vi "Main.vi"() -> ()   [LabVIEW 2019]
uses:
  <vilib>/myRIO/Common/Instrument Driver Framework/myRIO v1.0/UART/vis/myRIO v1.0 Close UART.vi
  <vilib>/Utility/error.llb/Error Cluster From Error Code.vi
  <vilib>/myRIO/Common/Instrument Driver Framework/Utilities/vis/FPGA Ref Manager.vi
  <vilib>/myRIO/Common/Instrument Driver Framework/myRIO v1.0/IRQ/vis/myRIO v1.0 IRQ Info FGV.vi
  <vilib>/myRIO/Common/Instrument Driver Framework/myRIO v1.0/IRQ/vis/myRIO v1.0 Timer IRQ Info FGV.vi
  <vilib>/myRIO/Instrument Drivers/Utilities/vis/Reset Index.vi
  <vilib>/myRIO/Common/Instrument Driver Framework/myRIO v1.0/Resource Manager/vis/myRIO v1.0 Block Write Resource Manager.vi
  <vilib>/myRIO/Instrument Drivers/Utilities/Utilities.lvlib
  <vilib>/myRIO/Instrument Drivers/Onboard IO/PWM/PWM.lvlib
panel:
  in  "BUKA":bool
  out "duty cycle [%]":dbl
  out "pulse width [ms]":dbl=1.5
  in  "freq [Hz]":dbl(slide)=50.0 scale=0.0..200.0
  in  "[ESC]":bool
  # "Servo Iris Mechanism"
  # "TUTUP"
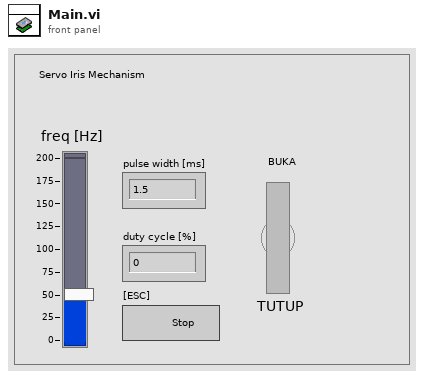
[diagram p1: front panel]
types:
  T1 = typedef "PWM.lvlib/PWM Reference.ctl" = cluster{"myRIO Reference":T2, "PWM Channels Enum":T6, "PWM Configuration":T7}
  T2 = typedef "myRIO Generic Hardware Reference.ctl" = cluster{"myRIO Model":T3, "myRIO Hardware Reference":T4}
  T3 = typedef "Hardware Version Enum.ctl" = enum16{"Unknown", "myRIO-1900", "myRIO-1950", "roboRIO", "NI ELVIS RIO CM", "ELVIS III"}
  T4 = typedef "myRIO v1.0 Reference.ctl" = cluster{"Generic FPGA Reference":T5, "Allow multiple opens":bool}
  T5 = typedef "Generic FPGA Reference.ctl" = refnum<k20>
  T6 = typedef "PWM Channels Enum.ctl" = enum16{"Not Connected", "C/PWM0", "C/PWM1", "A/PWM0", "A/PWM1", "A/PWM2", "A/PWM3", "A/PWM4", "A/PWM5", "A/PWM6", "A/PWM7", "A/PWM8", "A/PWM9", "A/PWM10", "A/PWM11", "A/PWM12", "A/PWM13", "A/PWM14", "A/PWM15", "A/PWM16", "A/PWM17", "A/PWM18", "A/PWM19", "B/PWM0", "B/PWM1", "B/PWM2", "B/PWM3", "B/PWM4", "B/PWM5", "B/PWM6", "B/PWM7", "B/PWM8", "B/PWM9", "B/PWM10", "B/PWM11", "B/PWM12", "B/PWM13", "B/PWM14", "B/PWM15", "B/PWM16", "B/PWM17", "B/PWM18", "B/PWM19", "PWM/PWM0", "PWM/PWM1", "PWM/PWM2", "PWM/PWM3", "PWM/PWM4", "PWM/PWM5", "PWM/PWM6", "PWM/PWM7", "PWM/PWM8", "PWM/PWM9"}
  T7 = typedef "PWM.lvlib/PWM Configuration.ctl" = cluster{"Frequency":dbl, "Duty Cycle":dbl}
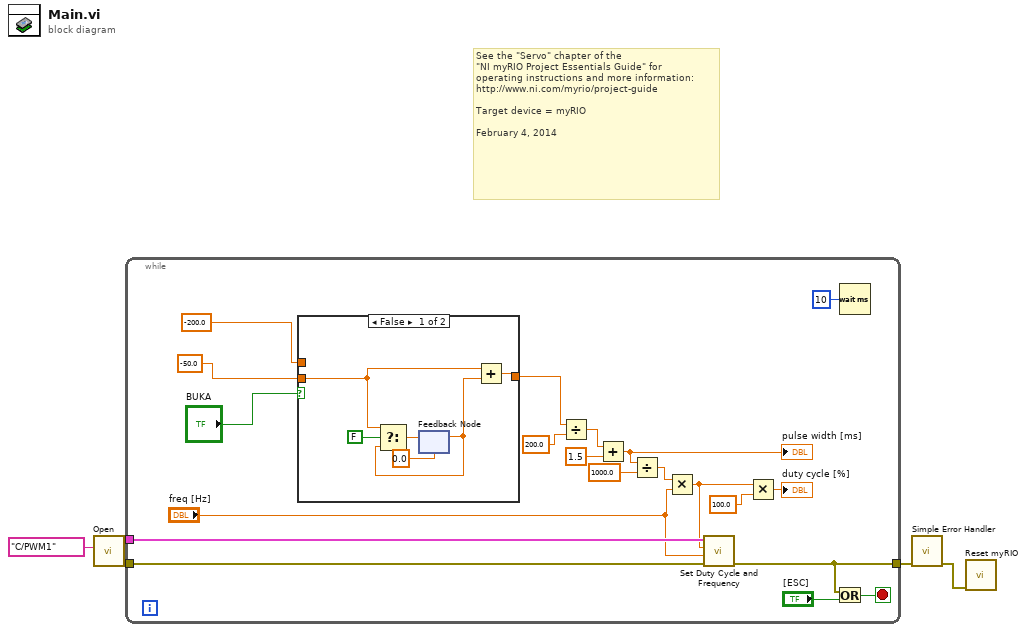
[diagram p0: block diagram]
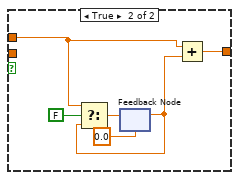
[diagram p2: hidden frame]
diagram:
  # "See the \"Servo\" chapter of the\n\"NI myRIO Project Essentials Guide\" for\noperating instructions and more information: \nhttp://www.ni.com/myrio/project-guide\n\nTarget device = myRIO\n\nFebruary 4, 2014"
  n1 = call <vilib>:"Open.vi"("Channel Name"=tag "C/PWM1") -> ("error out"=w3:errorcluster, "PWM Ref Out"=w4:T1)  [unwired: 9 in]
  n2 = while {
    tunnel: w4 -> [w17]
    tunnel: w3 -> [w16]
    tunnel: [w15] -> w2
    stop <- w25 stop-if-true
    n3 = case shown="False" "BUKA" {
      tunnel: -200.0 ("x") -> [_ w34]
      tunnel: -50.0 ("x") -> [w28 _]
      tunnel: [w26 w33] -> w6
      frame False {
        n4 = feedback #1(0.0 ("position [%FS]")) -> (w27:dbl)
        n5 = Select(t=w28, s=FALSE, f=w27) -> (s? t:f=w31:dbl)
        n6 = feedback-in #1(w31) -> ()
        n7 = Add(x=w28, y=w27) -> (x+y=w26:dbl)
      }
      frame True {
        n8 = feedback #2(0.0 ("position [%FS]")) -> (w32:dbl)
        n9 = Select(t=w34, s=FALSE, f=w32) -> (s? t:f=w37:dbl)
        n10 = feedback-in #2(w37) -> ()
        n11 = Add(x=w34, y=w32) -> (x+y=w33:dbl)
      }
    }
    n12 = Divide(x=w6, y=200.0) -> (x/y=w21:dbl)
    n13 = Add(x=w21, y=1.5) -> (x+y=w19:dbl)
    "pulse width [ms]" <- w19
    n14 = Divide(x=w19, y=1000.0) -> (x/y=w14:dbl)
    n15 = Multiply(x=w14, y="freq [Hz]") -> (x*y=w11:dbl)
    n16 = call <vilib>:"Set Duty Cycle and Frequency.vi"("error in (no error)"=w16, "Frequency [Hz]"="freq [Hz]", "Duty Cycle"=w11, "PWM Ref In"=w17) -> ("error out"=w15:errorcluster)  [unwired: 5 in, 1 out]
    n17 = Multiply(x=w11, y=100.0) -> (x*y=→"duty cycle [%]":dbl)
    n18 = Or(x=w15, y="[ESC]") -> (x .or. y?=w25:bool)
    n19 = Wait (ms)(milliseconds to wait=u32 10) -> ()  [unwired: 1 out]
  }
  n20 = call <vilib>:"Simple Error Handler.vi"("error in (no error)"=w2) -> ("error out"=w5:errorcluster)  [unwired: 4 in, 4 out]
  n21 = call <vilib>:"Reset myRIO.vi"("error in (no error)"=w5) -> ()  [unwired: 10 in, 1 out]
